vi "User Event to Name.vi"(0 "User Event":refnum<user-event>) -> (1 "Is Registered?":bool, 5 "Found?":bool, 6 "User Event Name":string)   [LabVIEW 2018, in "UserEvent.lvlib"]
uses:
  UserEvent.lvlib
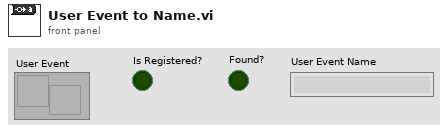
[diagram p1: front panel]
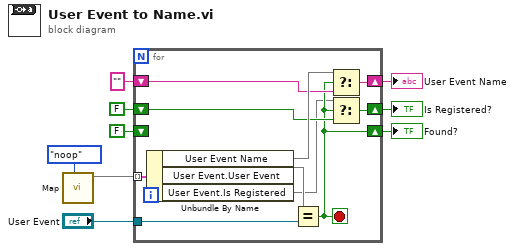
[diagram p0: block diagram]
diagram:
  n1 = call "Map.vi"("Action"=enum8{"noop", "get", "set", "pop"}."noop") -> (3:w8)  [unwired: 7 in, 3 out]
  n2 = for {
    tunnel: w8 -> [w19] mode=indexing
    tunnel: "User Event" -> [w17]
    shift-right: [w15] -> w4
    shift-left: "" ("User Event Name") -> [w14]
    shift-right: [w12] -> w3
    shift-left: FALSE -> [_]
    shift-right: [w10] -> w1
    shift-left: FALSE -> [w13]
    stop <- w12 stop-if-true
    n3 = Unbundle By Name(w19) -> ("User Event Name"=w16, "User Event.User Event"=w18, "User Event.Is Registered"=w11)
    n4 = Equal?(x=w18, y=w17) -> (x = y?=w12:bool)
    n5 = Select(t=w16, s=w12, f=w14) -> (s? t:f=w15:string)
    n6 = Select(t=w11, s=w12, f=w13) -> (s? t:f=w10:bool)
  }
  "User Event Name" <- w4
  "Found?" <- w3
  "Is Registered?" <- w1
